vi "SP_OEE_2_test.vi"() -> ()   [LabVIEW 2017] (continued)
                        n1245 = Decimal String To Number(string=w6823) -> (number=w6842:i32[])  [unwired: 2 in, 1 out]
                        n1246 = Decimal String To Number(string=w6824) -> (number=w6843:i32[])  [unwired: 2 in, 1 out]
                        n1247 = Decimal String To Number(string=w6825) -> (number=w6838:i32[])  [unwired: 2 in, 1 out]
                        n1248 = Compound Arithmetic op=ADD(w6815, w6813, w6811, w6809, w6807) -> (w6818:dbl[])
                        n1249 = Build Array(w6816) -> (w6837:string[][])
                        n1250 = Build Array(w6814) -> (w6836:string[][])
                        n1251 = Build Array(w6812) -> (w6835:string[][])
                        n1252 = Build Array(w6810) -> (w6834:string[][])
                        n1253 = Build Array(w6808) -> (w6833:string[][])
                        n1254 = Number To Fractional String(number=w6818, precision (6)=i16 2) -> (F-format string=w6817:string[])  [unwired: 2 in]
                        n1255 = Compound Arithmetic op=ADD(w6840, w6841, w6842, w6843, w6838) -> (w6844:i32[])
                        n1256 = Transpose 2D Array(2D array=w6837) -> (transposed array=w6831:string[][])
                        n1257 = Transpose 2D Array(2D array=w6836) -> (transposed array=w6830:string[][])
                        n1258 = Transpose 2D Array(2D array=w6835) -> (transposed array=w6829:string[][])
                        n1259 = Transpose 2D Array(2D array=w6834) -> (transposed array=w6828:string[][])
                        n1260 = Transpose 2D Array(2D array=w6833) -> (transposed array=w6827:string[][])
                        n1261 = Number To Decimal String(number=w6844) -> (decimal integer string=w6839:string[])  [unwired: 1 in]
                        n1262 = Build Array(w6817) -> (w6820:string[][])
                        n1263 = Transpose 2D Array(2D array=w6820) -> (transposed array=w6826:string[][])
                      }
                      frame #7 {
                        w6849 = string[] [""]
                        n1264 = Insert Into Array(array=w6857, index (col)=1 ("disabled index (col)"), new element #1=w6849, new element #2=w6849, new element #3=w6849, new element #4=w6849, new element #5=w6849, new element #6=w6849, new element #7=w6848, new element #8=w6847, new element #9=w6849, new element #10=w6849, new element #11=w6850, new element #12=w6851) -> (w6853:string[][])  [unwired: 1 in]
                        n1265 = call "flot graph for month n year.vi"("BD Date"=w6854, "error in (no error)"=w6856, "Count total"=w6850) -> ("error out"=w6855:errorcluster, "Run-Time Status"=w6852:cluster{"Array 2":timestamp[], dbl[]})  [unwired: 7 in]
                        n1266 = local write "Run-Time Status"(w6852) -> ()
                        n1267 = local write "Table"(w6853) -> ()
                      }
                    }
                  }
                  frame "2" {
                    n1268 = flat-sequence {
                      tunnel: w6869 -> [w6983]
                      tunnel: w6868 -> [w6981]
                      tunnel: [w6967] -> w6959
                      tunnel: [w6982] -> w6958
                      tunnel: w6867 -> [_]
                      tunnel: [w6986] -> w6957
                      tunnel: [w6966] -> w6956
                      tunnel: [w6965] -> w6955
                      tunnel: [w6964] -> w6954
                      tunnel: w6866 -> [w6966]
                      tunnel: w6865 -> [w6965]
                      tunnel: ["Where BREAKDOWN_DATE between '%s'and '%s' and BREAKDOWN_STK_HOLD_ID ='%d' and  SHIFT_ID = '%d' "] -> w6953
                      tunnel: [w6964] -> w6952
                      tunnel: w6864 -> [w6960]
                      tunnel: [w6960] -> w6863
                      tunnel: w6959 -> [w7047]
                      tunnel: w6958 -> [w7049]
                      tunnel: w6957 -> [w7045]
                      tunnel: w6956 -> [w7044]
                      tunnel: w6955 -> [w7043]
                      tunnel: [w7046] -> w6951
                      tunnel: [w7048] -> w6950
                      tunnel: [w7045] -> w6949
                      tunnel: [w7035] -> w6948
                      tunnel: [w7041] -> w6947
                      tunnel: [w7044] -> w6946
                      tunnel: [w7043] -> w6945
                      tunnel: w6954 -> [w7040]
                      tunnel: [w7040] -> w6944
                      tunnel: w6953 -> [w7037]
                      tunnel: [w7037] -> w6943
                      tunnel: [w7036] -> w6942
                      tunnel: w6952 -> [w7036]
                      tunnel: w6863 -> [w7034]
                      tunnel: [w7033] -> w6862
                      tunnel: w6951 -> [w7079]
                      tunnel: w6950 -> [w7077]
                      tunnel: w6949 -> [w7082]
                      tunnel: w6948 -> [w7081]
                      tunnel: w6947 -> [w7080]
                      tunnel: w6946 -> [w7075]
                      tunnel: w6945 -> [w7074]
                      tunnel: [w7082] -> w6941
                      tunnel: [w7081] -> w6940
                      tunnel: [w7080] -> w6939
                      tunnel: [w7078] -> w6938
                      tunnel: [w7072] -> w6937
                      tunnel: [w7071] -> w6936
                      tunnel: [w7076] -> w6935
                      tunnel: [w7075] -> w6934
                      tunnel: [w7074] -> w6933
                      tunnel: w6944 -> [w7070]
                      tunnel: [w7070] -> w6932
                      tunnel: w6943 -> [w7067]
                      tunnel: [w7067] -> w6931
                      tunnel: [w7066] -> w6930
                      tunnel: w6942 -> [w7066]
                      tunnel: w6862 -> [w7065]
                      tunnel: [w7064] -> w6861
                      tunnel: w6941 -> [w7117]
                      tunnel: w6940 -> [w7116]
                      tunnel: w6939 -> [w7115]
                      tunnel: w6938 -> [w7112]
                      tunnel: w6937 -> [w7114]
                      tunnel: w6936 -> [w7113]
                      tunnel: w6935 -> [w7110]
                      tunnel: w6934 -> [w7108]
                      tunnel: w6933 -> [w7107]
                      tunnel: [w7117] -> w6929
                      tunnel: [w7116] -> w6928
                      tunnel: [w7115] -> w6927
                      tunnel: [w7114] -> w6926
                      tunnel: [w7113] -> w6925
                      tunnel: [w7111] -> w6924
                      tunnel: [w7105] -> w6923
                      tunnel: [w7104] -> w6922
                      tunnel: [w7109] -> w6921
                      tunnel: [w7108] -> w6920
                      tunnel: [w7107] -> w6919
                      tunnel: w6932 -> [w7103]
                      tunnel: [w7103] -> w6918
                      tunnel: w6931 -> [w7100]
                      tunnel: [w7100] -> w6917
                      tunnel: [w7099] -> w6916
                      tunnel: w6930 -> [w7099]
                      tunnel: w6861 -> [w7098]
                      tunnel: [w7097] -> w6860
                      tunnel: w6929 -> [w7154]
                      tunnel: w6928 -> [w7153]
                      tunnel: w6927 -> [w7152]
                      tunnel: w6926 -> [w7151]
                      tunnel: w6925 -> [w7150]
                      tunnel: w6924 -> [w7147]
                      tunnel: w6923 -> [w7149]
                      tunnel: w6922 -> [w7148]
                      tunnel: w6921 -> [w7146]
                      tunnel: w6920 -> [w7143]
                      tunnel: w6919 -> [w7142]
                      tunnel: [w7154] -> w6915
                      tunnel: [w7153] -> w6914
                      tunnel: [w7152] -> w6913
                      tunnel: [w7151] -> w6912
                      tunnel: [w7150] -> w6911
                      tunnel: [w7149] -> w6910
                      tunnel: [w7148] -> w6909
                      tunnel: [w7145] -> w6908
                      tunnel: [w7144] -> w6907
                      tunnel: [w7140] -> w6906
                      tunnel: [w7139] -> w6905
                      tunnel: [w7143] -> w6904
                      tunnel: [w7142] -> w6903
                      tunnel: w6918 -> [w7138]
                      tunnel: [w7138] -> w6902
                      tunnel: w6917 -> [w7135]
                      tunnel: [w7135] -> w6901
                      tunnel: [w7134] -> w6900
                      tunnel: w6916 -> [w7134]
                      tunnel: w6860 -> [w7132]
                      tunnel: w6915 -> [w7177]
                      tunnel: w6914 -> [w7176]
                      tunnel: w6913 -> [w7175]
                      tunnel: w6912 -> [w7174]
                      tunnel: w6911 -> [w7173]
                      tunnel: w6910 -> [w7172]
                      tunnel: w6909 -> [w7171]
                      tunnel: w6908 -> [w7166]
                      tunnel: w6907 -> [w7168]
                      tunnel: w6906 -> [w7170]
                      tunnel: w6905 -> [w7169]
                      tunnel: w6904 -> [w7163]
                      tunnel: w6903 -> [w7164]
                      tunnel: [w7177] -> w6899
                      tunnel: [w7176] -> w6898
                      tunnel: [w7175] -> w6897
                      tunnel: [w7174] -> w6896
                      tunnel: [w7173] -> w6895
                      tunnel: [w7172] -> w6894
                      tunnel: [w7171] -> w6893
                      tunnel: [w7170] -> w6892
                      tunnel: [w7169] -> w6891
                      tunnel: [w7167] -> w6890
                      tunnel: [w7165] -> w6889
                      tunnel: [w7161] -> w6888
                      tunnel: [w7159] -> w6887
                      tunnel: w6902 -> [w7160]
                      tunnel: w6901 -> [w7156]
                      tunnel: [w7155] -> w6886
                      tunnel: w6900 -> [w7155]
                      tunnel: w6899 -> [w7216]
                      tunnel: w6898 -> [w7209]
                      tunnel: w6897 -> [w7200]
                      tunnel: w6896 -> [w7208]
                      tunnel: w6895 -> [w7198]
                      tunnel: w6894 -> [w7207]
                      tunnel: w6893 -> [w7196]
                      tunnel: w6892 -> [w7206]
                      tunnel: w6891 -> [w7194]
                      tunnel: w6890 -> [w7230]
                      tunnel: w6889 -> [w7229]
                      tunnel: w6888 -> [w7205]
                      tunnel: w6887 -> [w7192]
                      tunnel: [w7230] -> w6885
                      tunnel: [w7229] -> w6884
                      tunnel: [w7223] -> w6883
                      tunnel: [w7216] -> w6882
                      tunnel: [w7215] -> w6881
                      tunnel: [w7214] -> w6880
                      tunnel: [w7213] -> w6879
                      tunnel: [w7212] -> w6878
                      tunnel: [w7211] -> w6877
                      tunnel: [w7210] -> w6876
                      tunnel: [w7209] -> w6875
                      tunnel: [w7208] -> w6874
                      tunnel: [w7207] -> w6873
                      tunnel: [w7206] -> w6872
                      tunnel: [w7205] -> w6871
                      tunnel: [w7190] -> w6870
                      tunnel: w6886 -> [w7190]
                      tunnel: [w7243] -> _
                      tunnel: [w7239] -> _
                      tunnel: w6885 -> [w7240]
                      tunnel: w6884 -> [w7243]
                      tunnel: w6883 -> [w7234]
                      tunnel: w6882 -> [w7241]
                      tunnel: w6881 -> [_]
                      tunnel: w6880 -> [_]
                      tunnel: w6879 -> [_]
                      tunnel: w6878 -> [w7231]
                      tunnel: w6877 -> [_]
                      tunnel: w6876 -> [w7235]
                      tunnel: w6875 -> [_]
                      tunnel: w6874 -> [_]
                      tunnel: w6873 -> [_]
                      tunnel: w6872 -> [w7232]
                      tunnel: w6871 -> [_]
                      tunnel: w6870 -> [w7238]
                      frame #0 {
                        w6974 = "%Y-%m-%d" ("time format string (%c)")
                        n1269 = Decimal String To Number(string=w6960) -> (number=w6961:i32)  [unwired: 2 in, 1 out]
                        n1270 = property on="Table" class="Tbl (strict)"("Visible"=TRUE) -> ()  [unwired: 2 in, 2 out]
                        n1271 = Format Date/Time String(time format string (%c)=w6974, seconds (now)=w6966) -> (date/time string=w6975:string)  [unwired: 1 in]
                        n1272 = Format Date/Time String(time format string (%c)=w6974, seconds (now)=w6965) -> (date/time string=w6973:string)  [unwired: 1 in]
                        n1273 = Format Into String(format string="Where BREAKDOWN_DATE between '%s' and '%s' and  SHIFT_ID = '%d'  ", w6975, w6973, w6961) -> (resulting string=w6972:string)  [unwired: 2 in, 1 out]
                        n1274 = call <vilib>:"DB Tools Select Data.vi"("condition"=w6972, "error in (no error)"=w6981, "columns"=string[] ["BREAKDOWN_DATE"], "table"="STATION_1_LOG_HISTORY", "connection reference"=w6983) -> ("error out"=w6968:errorcluster, "data"=w6971:variant[][], "connection reference out"=w6982:T2)  [unwired: 1 in]
                        n1275 = property on="Table 2" class="Tbl (strict)"("Visible"=FALSE) -> ()  [unwired: 2 in, 2 out]
                        n1276 = xnode "Database Variant To Data"("database variant"=w6971, "error in (no error)"=w6968, "type"=string[][] [] ("Elements Found")) -> ("data"=w6969:string[][], "error out"=w6967:errorcluster)
                        n1277 = Index Array(array=w6969, index (col)=0 ("disabled index (col)")) -> (element=w6977:string[])  [unwired: 1 in]
                        n1278 = call "Search_1d_array_element.vi"("Count in"=string[] [] ("Elements Found"), "BD Date"=w6977, "Elements Found in"=string[] [] ("Elements Found")) -> ("Elements Found out"=w6964:string[])  [unwired: 4 in, 2 out]
                        n1279 = Build Array(w6964) -> (w6987:string[][])
                        n1280 = Transpose 2D Array(2D array=w6987) -> (transposed array=w6986:string[][])
                      }
                      frame #1 {
                        n1281 = disable-structure shown="Enabled" {
                          disable-tunnel: w7049 -> [w7060 w7062]
                          disable-tunnel: [w7059 w7062] -> w7048
                          disable-tunnel: w7047 -> [w7058 w7063]
                          disable-tunnel: [w7057 w7063] -> w7046
                          disable-tunnel: w7044 -> [w7055 _]
                          disable-tunnel: w7043 -> [w7054 _]
                          disable-tunnel: [w7053 _] -> w7042
                          disable-tunnel: [w7052 _] -> w7039
                          disable-tunnel: w7037 -> [w7051 _]
                          disable-tunnel: w7034 -> [w7050 w7061]
                          disable-tunnel: [_ w7061] -> w7033
                          frame Disabled {
                            n1282 = call "Stack_holderwise_total_bd_count_&_duration_2.vi"("Refnum in"=w7060, "BREAKDOWN_STK_HOLD_ID"=1, "condition"=w7051, "Form Date"=w7055, "To Date"=w7054, "error in (no error)"=w7058, "Shift"=w7050) -> ("Refnum out"=w7059:T2, "Count out"=w7053:string[], "appended array"=w7052:dbl[], "error out"=w7057:errorcluster)  [unwired: 5 in]
                          }
                          frame Enabled {
                          }
                        }
                        n1283 = call "NUMERIC TO STRING.vi"("appended array"=w7039) -> ("Array"=w7038:string[])  [unwired: 4 in]
                        n1284 = call "Insert_empty_element_with_zero.vi"("searched date"=w7042, "fixed date"=w7040) -> ("O/P"=w7035:string[])  [unwired: 9 in]
                        n1285 = call "Insert_empty_element_with_zero.vi"("searched date"=w7038, "fixed date"=w7040) -> ("O/P"=w7041:string[])  [unwired: 9 in]
                      }
                      frame #2 {
                        n1286 = disable-structure shown="Enabled" {
                          disable-tunnel: w7079 -> [w7093 w7095]
                          disable-tunnel: [w7092 w7095] -> w7078
                          disable-tunnel: w7077 -> [w7091 w7096]
                          disable-tunnel: [w7090 w7096] -> w7076
                          disable-tunnel: w7075 -> [w7089 _]
                          disable-tunnel: w7074 -> [w7088 _]
                          disable-tunnel: [w7087 _] -> w7073
                          disable-tunnel: [w7086 _] -> w7069
                          disable-tunnel: w7067 -> [w7085 _]
                          disable-tunnel: w7065 -> [w7083 w7094]
                          disable-tunnel: [_ w7094] -> w7064
                          frame Disabled {
                            n1287 = call "Stack_holderwise_total_bd_count_&_duration_2.vi"("Refnum in"=w7091, "BREAKDOWN_STK_HOLD_ID"=2, "condition"=w7085, "Form Date"=w7089, "To Date"=w7088, "error in (no error)"=w7093, "Shift"=w7083) -> ("Refnum out"=w7090:T2, "Count out"=w7087:string[], "appended array"=w7086:dbl[], "error out"=w7092:errorcluster)  [unwired: 5 in]
                          }
                          frame Enabled {
                          }
                        }
                        n1288 = call "Insert_empty_element_with_zero.vi"("searched date"=w7073, "fixed date"=w7070) -> ("O/P"=w7072:string[])  [unwired: 9 in]
                        n1289 = call "NUMERIC TO STRING.vi"("appended array"=w7069) -> ("Array"=w7068:string[])  [unwired: 4 in]
                        n1290 = call "Insert_empty_element_with_zero.vi"("searched date"=w7068, "fixed date"=w7070) -> ("O/P"=w7071:string[])  [unwired: 9 in]
                      }
                      frame #3 {
                        n1291 = disable-structure shown="Enabled" {
                          disable-tunnel: w7112 -> [w7128 w7130]
                          disable-tunnel: [w7127 w7130] -> w7111
                          disable-tunnel: w7110 -> [w7126 w7131]
                          disable-tunnel: [w7125 w7131] -> w7109
                          disable-tunnel: w7108 -> [w7124 _]
                          disable-tunnel: w7107 -> [w7123 _]
                          disable-tunnel: [w7122 _] -> w7106
                          disable-tunnel: [w7121 _] -> w7102
                          disable-tunnel: w7100 -> [w7120 _]
                          disable-tunnel: w7098 -> [w7118 w7129]
                          disable-tunnel: [_ w7129] -> w7097
                          frame Disabled {
                            n1292 = call "Stack_holderwise_total_bd_count_&_duration_2.vi"("Refnum in"=w7126, "BREAKDOWN_STK_HOLD_ID"=3, "condition"=w7120, "Form Date"=w7124, "To Date"=w7123, "error in (no error)"=w7128, "Shift"=w7118) -> ("Refnum out"=w7125:T2, "Count out"=w7122:string[], "appended array"=w7121:dbl[], "error out"=w7127:errorcluster)  [unwired: 5 in]
                          }
                          frame Enabled {
                          }
                        }
                        n1293 = call "Insert_empty_element_with_zero.vi"("searched date"=w7106, "fixed date"=w7103) -> ("O/P"=w7105:string[])  [unwired: 9 in]
                        n1294 = call "NUMERIC TO STRING.vi"("appended array"=w7102) -> ("Array"=w7101:string[])  [unwired: 4 in]
                        n1295 = call "Insert_empty_element_with_zero.vi"("searched date"=w7101, "fixed date"=w7103) -> ("O/P"=w7104:string[])  [unwired: 9 in]
                      }
                      frame #4 {
                        n1296 = call "Stack_holderwise_total_bd_count_&_duration_2.vi"("Refnum in"=w7146, "BREAKDOWN_STK_HOLD_ID"=4, "condition"=w7135, "Form Date"=w7143, "To Date"=w7142, "error in (no error)"=w7147, "Shift"=w7132) -> ("Refnum out"=w7145:T2, "Count out"=w7141:string[], "appended array"=w7137:dbl[], "error out"=w7144:errorcluster)  [unwired: 5 in]
                        n1297 = call "Insert_empty_element_with_zero.vi"("searched date"=w7141, "fixed date"=w7138) -> ("O/P"=w7140:string[])  [unwired: 9 in]
                        n1298 = call "NUMERIC TO STRING.vi"("appended array"=w7137) -> ("Array"=w7136:string[])  [unwired: 4 in]
                        n1299 = call "Insert_empty_element_with_zero.vi"("searched date"=w7136, "fixed date"=w7138) -> ("O/P"=w7139:string[])  [unwired: 9 in]
                      }
                      frame #5 {
                        n1300 = disable-structure shown="Enabled" {
                          disable-tunnel: w7168 -> [w7186 w7189]
                          disable-tunnel: [w7185 w7189] -> w7167
                          disable-tunnel: w7166 -> [w7184 w7188]
                          disable-tunnel: [w7183 w7188] -> w7165
                          disable-tunnel: w7164 -> [w7182 _]
                          disable-tunnel: w7163 -> [w7181 _]
                          disable-tunnel: [w7180 _] -> w7162
                          disable-tunnel: [w7179 _] -> w7158
                          disable-tunnel: w7156 -> [w7178 _]
                          frame Disabled {
                            n1301 = call "Stack_holderwise_total_bd_count_&_duration.vi"("Refnum in"=w7184, "BREAKDOWN_STK_HOLD_ID"=5, "condition"=w7178, "Form Date"=w7181, "To Date"=w7182, "error in (no error)"=w7186) -> ("Refnum out"=w7183:T2, "Count out"=w7180:string[], "appended array"=w7179:dbl[], "error out"=w7185:errorcluster)  [unwired: 6 in]
                          }
                          frame Enabled {
                          }
                        }
                        n1302 = call "NUMERIC TO STRING.vi"("appended array"=w7158) -> ("Array"=w7157:string[])  [unwired: 4 in]
                        n1303 = call "Insert_empty_element_with_zero.vi"("searched date"=w7162, "fixed date"=w7160) -> ("O/P"=w7161:string[])  [unwired: 9 in]
                        n1304 = call "Insert_empty_element_with_zero.vi"("searched date"=w7157, "fixed date"=w7160) -> ("O/P"=w7159:string[])  [unwired: 9 in]
                      }
                      frame #6 {
                        n1305 = call "String to numeric.vi"("Array"=w7200) -> ("Array 2"=w7199:dbl[])  [unwired: 4 in]
                        n1306 = call "String to numeric.vi"("Array"=w7198) -> ("Array 2"=w7197:dbl[])  [unwired: 4 in]
                        n1307 = call "String to numeric.vi"("Array"=w7196) -> ("Array 2"=w7195:dbl[])  [unwired: 4 in]
                        n1308 = call "String to numeric.vi"("Array"=w7194) -> ("Array 2"=w7193:dbl[])  [unwired: 4 in]
                        n1309 = call "String to numeric.vi"("Array"=w7192) -> ("Array 2"=w7191:dbl[])  [unwired: 4 in]
                        n1310 = Decimal String To Number(string=w7205) -> (number=w7224:i32[])  [unwired: 2 in, 1 out]
                        n1311 = Decimal String To Number(string=w7206) -> (number=w7225:i32[])  [unwired: 2 in, 1 out]
                        n1312 = Decimal String To Number(string=w7207) -> (number=w7226:i32[])  [unwired: 2 in, 1 out]
                        n1313 = Decimal String To Number(string=w7208) -> (number=w7227:i32[])  [unwired: 2 in, 1 out]
                        n1314 = Decimal String To Number(string=w7209) -> (number=w7222:i32[])  [unwired: 2 in, 1 out]
                        n1315 = Compound Arithmetic op=ADD(w7199, w7197, w7195, w7193, w7191) -> (w7202:dbl[])
                        n1316 = Build Array(w7200) -> (w7221:string[][])
                        n1317 = Build Array(w7198) -> (w7220:string[][])
                        n1318 = Build Array(w7196) -> (w7219:string[][])
                        n1319 = Build Array(w7194) -> (w7218:string[][])
                        n1320 = Build Array(w7192) -> (w7217:string[][])
                        n1321 = Number To Fractional String(number=w7202, precision (6)=i16 2) -> (F-format string=w7201:string[])  [unwired: 2 in]
                        n1322 = Compound Arithmetic op=ADD(w7224, w7225, w7226, w7227, w7222) -> (w7228:i32[])
                        n1323 = Transpose 2D Array(2D array=w7221) -> (transposed array=w7215:string[][])
                        n1324 = Transpose 2D Array(2D array=w7220) -> (transposed array=w7214:string[][])
                        n1325 = Transpose 2D Array(2D array=w7219) -> (transposed array=w7213:string[][])
                        n1326 = Transpose 2D Array(2D array=w7218) -> (transposed array=w7212:string[][])
                        n1327 = Transpose 2D Array(2D array=w7217) -> (transposed array=w7211:string[][])
                        n1328 = Number To Decimal String(number=w7228) -> (decimal integer string=w7223:string[])  [unwired: 1 in]
                        n1329 = Build Array(w7201) -> (w7204:string[][])
                        n1330 = Transpose 2D Array(2D array=w7204) -> (transposed array=w7210:string[][])
                      }
                      frame #7 {
                        w7233 = string[] [""]
                        n1331 = Insert Into Array(array=w7241, index (col)=1 ("disabled index (col)"), new element #1=w7233, new element #2=w7233, new element #3=w7233, new element #4=w7233, new element #5=w7233, new element #6=w7233, new element #7=w7232, new element #8=w7231, new element #9=w7233, new element #10=w7233, new element #11=w7234, new element #12=w7235) -> (w7237:string[][])  [unwired: 1 in]
                        n1332 = call "flot graph for month n year.vi"("BD Date"=w7238, "error in (no error)"=w7240, "Count total"=w7234) -> ("error out"=w7239:errorcluster, "Run-Time Status"=w7236:cluster{"Array 2":timestamp[], dbl[]})  [unwired: 7 in]
                        n1333 = local write "Run-Time Status"(w7236) -> ()
                        n1334 = local write "Table"(w7237) -> ()
                      }
                    }
                  }
                  frame "3" {
                    n1335 = flat-sequence {
                      tunnel: w7253 -> [w7367]
                      tunnel: w7252 -> [w7365]
                      tunnel: [w7351] -> w7343
                      tunnel: [w7366] -> w7342
                      tunnel: w7251 -> [_]
                      tunnel: [w7370] -> w7341
                      tunnel: [w7350] -> w7340
                      tunnel: [w7349] -> w7339
                      tunnel: [w7348] -> w7338
                      tunnel: w7250 -> [w7350]
                      tunnel: w7249 -> [w7349]
                      tunnel: ["Where BREAKDOWN_DATE between '%s'and '%s' and BREAKDOWN_STK_HOLD_ID ='%d' and  SHIFT_ID = '%d' "] -> w7337
                      tunnel: [w7348] -> w7336
                      tunnel: w7248 -> [w7344]
                      tunnel: [w7344] -> w7247
                      tunnel: w7343 -> [w7431]
                      tunnel: w7342 -> [w7433]
                      tunnel: w7341 -> [w7429]
                      tunnel: w7340 -> [w7428]
                      tunnel: w7339 -> [w7427]
                      tunnel: [w7430] -> w7335
                      tunnel: [w7432] -> w7334
                      tunnel: [w7429] -> w7333
                      tunnel: [w7419] -> w7332
                      tunnel: [w7425] -> w7331
                      tunnel: [w7428] -> w7330
                      tunnel: [w7427] -> w7329
                      tunnel: w7338 -> [w7424]
                      tunnel: [w7424] -> w7328
                      tunnel: w7337 -> [w7421]
                      tunnel: [w7421] -> w7327
                      tunnel: [w7420] -> w7326
                      tunnel: w7336 -> [w7420]
                      tunnel: w7247 -> [w7418]
                      tunnel: [w7417] -> w7246
                      tunnel: w7335 -> [w7463]
                      tunnel: w7334 -> [w7461]
                      tunnel: w7333 -> [w7466]
                      tunnel: w7332 -> [w7465]
                      tunnel: w7331 -> [w7464]
                      tunnel: w7330 -> [w7459]
                      tunnel: w7329 -> [w7458]
                      tunnel: [w7466] -> w7325
                      tunnel: [w7465] -> w7324
                      tunnel: [w7464] -> w7323
                      tunnel: [w7462] -> w7322
                      tunnel: [w7456] -> w7321
                      tunnel: [w7455] -> w7320
                      tunnel: [w7460] -> w7319
                      tunnel: [w7459] -> w7318
                      tunnel: [w7458] -> w7317
                      tunnel: w7328 -> [w7454]
                      tunnel: [w7454] -> w7316
                      tunnel: w7327 -> [w7451]
                      tunnel: [w7451] -> w7315
                      tunnel: [w7450] -> w7314
                      tunnel: w7326 -> [w7450]
                      tunnel: w7246 -> [w7449]
                      tunnel: [w7448] -> w7245
                      tunnel: w7325 -> [w7501]
                      tunnel: w7324 -> [w7500]
                      tunnel: w7323 -> [w7499]
                      tunnel: w7322 -> [w7496]
                      tunnel: w7321 -> [w7498]
                      tunnel: w7320 -> [w7497]
                      tunnel: w7319 -> [w7494]
                      tunnel: w7318 -> [w7492]
                      tunnel: w7317 -> [w7491]
                      tunnel: [w7501] -> w7313
                      tunnel: [w7500] -> w7312
                      tunnel: [w7499] -> w7311
                      tunnel: [w7498] -> w7310
                      tunnel: [w7497] -> w7309
                      tunnel: [w7495] -> w7308
                      tunnel: [w7489] -> w7307
                      tunnel: [w7488] -> w7306
                      tunnel: [w7493] -> w7305
                      tunnel: [w7492] -> w7304
                      tunnel: [w7491] -> w7303
                      tunnel: w7316 -> [w7487]
                      tunnel: [w7487] -> w7302
                      tunnel: w7315 -> [w7484]
                      tunnel: [w7484] -> w7301
                      tunnel: [w7483] -> w7300
                      tunnel: w7314 -> [w7483]
                      tunnel: w7245 -> [w7482]
                      tunnel: [w7481] -> w7244
                      tunnel: w7313 -> [w7538]
                      tunnel: w7312 -> [w7537]
                      tunnel: w7311 -> [w7536]
                      tunnel: w7310 -> [w7535]
                      tunnel: w7309 -> [w7534]
                      tunnel: w7308 -> [w7531]
                      tunnel: w7307 -> [w7533]
                      tunnel: w7306 -> [w7532]
                      tunnel: w7305 -> [w7530]
                      tunnel: w7304 -> [w7527]
                      tunnel: w7303 -> [w7526]
                      tunnel: [w7538] -> w7299
                      tunnel: [w7537] -> w7298
                      tunnel: [w7536] -> w7297
                      tunnel: [w7535] -> w7296
                      tunnel: [w7534] -> w7295
                      tunnel: [w7533] -> w7294
                      tunnel: [w7532] -> w7293
                      tunnel: [w7529] -> w7292
                      tunnel: [w7528] -> w7291
                      tunnel: [w7524] -> w7290
                      tunnel: [w7523] -> w7289
                      tunnel: [w7527] -> w7288
                      tunnel: [w7526] -> w7287
                      tunnel: w7302 -> [w7522]
                      tunnel: [w7522] -> w7286
                      tunnel: w7301 -> [w7519]
                      tunnel: [w7519] -> w7285
                      tunnel: [w7518] -> w7284
                      tunnel: w7300 -> [w7518]
                      tunnel: w7244 -> [w7516]
                      tunnel: w7299 -> [w7561]
                      tunnel: w7298 -> [w7560]
                      tunnel: w7297 -> [w7559]
                      tunnel: w7296 -> [w7558]
                      tunnel: w7295 -> [w7557]
                      tunnel: w7294 -> [w7556]
                      tunnel: w7293 -> [w7555]
                      tunnel: w7292 -> [w7550]
                      tunnel: w7291 -> [w7552]
                      tunnel: w7290 -> [w7554]
                      tunnel: w7289 -> [w7553]
                      tunnel: w7288 -> [w7547]
                      tunnel: w7287 -> [w7548]
                      tunnel: [w7561] -> w7283
                      tunnel: [w7560] -> w7282
                      tunnel: [w7559] -> w7281
                      tunnel: [w7558] -> w7280
                      tunnel: [w7557] -> w7279
                      tunnel: [w7556] -> w7278
                      tunnel: [w7555] -> w7277
                      tunnel: [w7554] -> w7276
                      tunnel: [w7553] -> w7275
                      tunnel: [w7551] -> w7274
                      tunnel: [w7549] -> w7273
                      tunnel: [w7545] -> w7272
                      tunnel: [w7543] -> w7271
                      tunnel: w7286 -> [w7544]
                      tunnel: w7285 -> [w7540]
                      tunnel: [w7539] -> w7270
                      tunnel: w7284 -> [w7539]
                      tunnel: w7283 -> [w7600]
                      tunnel: w7282 -> [w7593]
                      tunnel: w7281 -> [w7584]
                      tunnel: w7280 -> [w7592]
                      tunnel: w7279 -> [w7582]
                      tunnel: w7278 -> [w7591]
                      tunnel: w7277 -> [w7580]
                      tunnel: w7276 -> [w7590]
                      tunnel: w7275 -> [w7578]
                      tunnel: w7274 -> [w7614]
                      tunnel: w7273 -> [w7613]
                      tunnel: w7272 -> [w7589]
                      tunnel: w7271 -> [w7576]
                      tunnel: [w7614] -> w7269
                      tunnel: [w7613] -> w7268
                      tunnel: [w7607] -> w7267
                      tunnel: [w7600] -> w7266
                      tunnel: [w7599] -> w7265
                      tunnel: [w7598] -> w7264
                      tunnel: [w7597] -> w7263
                      tunnel: [w7596] -> w7262
                      tunnel: [w7595] -> w7261
                      tunnel: [w7594] -> w7260
                      tunnel: [w7593] -> w7259
                      tunnel: [w7592] -> w7258
                      tunnel: [w7591] -> w7257
                      tunnel: [w7590] -> w7256
                      tunnel: [w7589] -> w7255
                      tunnel: [w7574] -> w7254
                      tunnel: w7270 -> [w7574]
                      tunnel: [w7627] -> _
                      tunnel: [w7623] -> _
                      tunnel: w7269 -> [w7624]
                      tunnel: w7268 -> [w7627]
                      tunnel: w7267 -> [w7618]
                      tunnel: w7266 -> [w7625]
                      tunnel: w7265 -> [_]
                      tunnel: w7264 -> [_]
                      tunnel: w7263 -> [_]
                      tunnel: w7262 -> [w7615]
                      tunnel: w7261 -> [_]
                      tunnel: w7260 -> [w7619]
                      tunnel: w7259 -> [_]
                      tunnel: w7258 -> [_]
                      tunnel: w7257 -> [_]
                      tunnel: w7256 -> [w7616]
                      tunnel: w7255 -> [_]
                      tunnel: w7254 -> [w7622]
                      frame #0 {
                        w7358 = "%Y-%m-%d" ("time format string (%c)")
                        n1336 = Decimal String To Number(string=w7344) -> (number=w7345:i32)  [unwired: 2 in, 1 out]
                        n1337 = property on="Table" class="Tbl (strict)"("Visible"=TRUE) -> ()  [unwired: 2 in, 2 out]
                        n1338 = Format Date/Time String(time format string (%c)=w7358, seconds (now)=w7350) -> (date/time string=w7359:string)  [unwired: 1 in]
                        n1339 = Format Date/Time String(time format string (%c)=w7358, seconds (now)=w7349) -> (date/time string=w7357:string)  [unwired: 1 in]
                        n1340 = Format Into String(format string="Where BREAKDOWN_DATE between '%s' and '%s' and  SHIFT_ID = '%d'  ", w7359, w7357, w7345) -> (resulting string=w7356:string)  [unwired: 2 in, 1 out]
                        n1341 = call <vilib>:"DB Tools Select Data.vi"("condition"=w7356, "error in (no error)"=w7365, "columns"=string[] ["BREAKDOWN_DATE"], "table"="STATION_1_LOG_HISTORY", "connection reference"=w7367) -> ("error out"=w7352:errorcluster, "data"=w7355:variant[][], "connection reference out"=w7366:T2)  [unwired: 1 in]
                        n1342 = property on="Table 2" class="Tbl (strict)"("Visible"=FALSE) -> ()  [unwired: 2 in, 2 out]
                        n1343 = xnode "Database Variant To Data"("database variant"=w7355, "error in (no error)"=w7352, "type"=string[][] [] ("Elements Found")) -> ("data"=w7353:string[][], "error out"=w7351:errorcluster)
                        n1344 = Index Array(array=w7353, index (col)=0 ("disabled index (col)")) -> (element=w7361:string[])  [unwired: 1 in]
                        n1345 = call "Search_1d_array_element.vi"("Count in"=string[] [] ("Elements Found"), "BD Date"=w7361, "Elements Found in"=string[] [] ("Elements Found")) -> ("Elements Found out"=w7348:string[])  [unwired: 4 in, 2 out]
                        n1346 = Build Array(w7348) -> (w7371:string[][])
                        n1347 = Transpose 2D Array(2D array=w7371) -> (transposed array=w7370:string[][])
                      }
                      frame #1 {
                        n1348 = disable-structure shown="Enabled" {
                          disable-tunnel: w7433 -> [w7444 w7446]
                          disable-tunnel: [w7443 w7446] -> w7432
                          disable-tunnel: w7431 -> [w7442 w7447]
                          disable-tunnel: [w7441 w7447] -> w7430
                          disable-tunnel: w7428 -> [w7439 _]
                          disable-tunnel: w7427 -> [w7438 _]
                          disable-tunnel: [w7437 _] -> w7426
                          disable-tunnel: [w7436 _] -> w7423
                          disable-tunnel: w7421 -> [w7435 _]
                          disable-tunnel: w7418 -> [w7434 w7445]
                          disable-tunnel: [_ w7445] -> w7417
                          frame Disabled {
                            n1349 = call "Stack_holderwise_total_bd_count_&_duration_2.vi"("Refnum in"=w7444, "BREAKDOWN_STK_HOLD_ID"=1, "condition"=w7435, "Form Date"=w7439, "To Date"=w7438, "error in (no error)"=w7442, "Shift"=w7434) -> ("Refnum out"=w7443:T2, "Count out"=w7437:string[], "appended array"=w7436:dbl[], "error out"=w7441:errorcluster)  [unwired: 5 in]
                          }
                          frame Enabled {
                          }
                        }
                        n1350 = call "NUMERIC TO STRING.vi"("appended array"=w7423) -> ("Array"=w7422:string[])  [unwired: 4 in]
                        n1351 = call "Insert_empty_element_with_zero.vi"("searched date"=w7426, "fixed date"=w7424) -> ("O/P"=w7419:string[])  [unwired: 9 in]
                        n1352 = call "Insert_empty_element_with_zero.vi"("searched date"=w7422, "fixed date"=w7424) -> ("O/P"=w7425:string[])  [unwired: 9 in]
                      }
                      frame #2 {
                        n1353 = disable-structure shown="Enabled" {
                          disable-tunnel: w7463 -> [w7477 w7479]
                          disable-tunnel: [w7476 w7479] -> w7462
                          disable-tunnel: w7461 -> [w7475 w7480]
                          disable-tunnel: [w7474 w7480] -> w7460
                          disable-tunnel: w7459 -> [w7473 _]
                          disable-tunnel: w7458 -> [w7472 _]
                          disable-tunnel: [w7471 _] -> w7457
                          disable-tunnel: [w7470 _] -> w7453
                          disable-tunnel: w7451 -> [w7469 _]
                          disable-tunnel: w7449 -> [w7467 w7478]
                          disable-tunnel: [_ w7478] -> w7448
                          frame Disabled {
                            n1354 = call "Stack_holderwise_total_bd_count_&_duration_2.vi"("Refnum in"=w7475, "BREAKDOWN_STK_HOLD_ID"=2, "condition"=w7469, "Form Date"=w7473, "To Date"=w7472, "error in (no error)"=w7477, "Shift"=w7467) -> ("Refnum out"=w7474:T2, "Count out"=w7471:string[], "appended array"=w7470:dbl[], "error out"=w7476:errorcluster)  [unwired: 5 in]
                          }
                          frame Enabled {
                          }
                        }
                        n1355 = call "Insert_empty_element_with_zero.vi"("searched date"=w7457, "fixed date"=w7454) -> ("O/P"=w7456:string[])  [unwired: 9 in]
                        n1356 = call "NUMERIC TO STRING.vi"("appended array"=w7453) -> ("Array"=w7452:string[])  [unwired: 4 in]
                        n1357 = call "Insert_empty_element_with_zero.vi"("searched date"=w7452, "fixed date"=w7454) -> ("O/P"=w7455:string[])  [unwired: 9 in]
                      }
                      frame #3 {
                        n1358 = disable-structure shown="Enabled" {
                          disable-tunnel: w7496 -> [w7512 w7514]
                          disable-tunnel: [w7511 w7514] -> w7495
                          disable-tunnel: w7494 -> [w7510 w7515]
                          disable-tunnel: [w7509 w7515] -> w7493
                          disable-tunnel: w7492 -> [w7508 _]
                          disable-tunnel: w7491 -> [w7507 _]
                          disable-tunnel: [w7506 _] -> w7490
                          disable-tunnel: [w7505 _] -> w7486
                          disable-tunnel: w7484 -> [w7504 _]
                          disable-tunnel: w7482 -> [w7502 w7513]
                          disable-tunnel: [_ w7513] -> w7481
                          frame Disabled {
                            n1359 = call "Stack_holderwise_total_bd_count_&_duration_2.vi"("Refnum in"=w7510, "BREAKDOWN_STK_HOLD_ID"=3, "condition"=w7504, "Form Date"=w7508, "To Date"=w7507, "error in (no error)"=w7512, "Shift"=w7502) -> ("Refnum out"=w7509:T2, "Count out"=w7506:string[], "appended array"=w7505:dbl[], "error out"=w7511:errorcluster)  [unwired: 5 in]
                          }
                          frame Enabled {
                          }
                        }
                        n1360 = call "Insert_empty_element_with_zero.vi"("searched date"=w7490, "fixed date"=w7487) -> ("O/P"=w7489:string[])  [unwired: 9 in]
                        n1361 = call "NUMERIC TO STRING.vi"("appended array"=w7486) -> ("Array"=w7485:string[])  [unwired: 4 in]
                        n1362 = call "Insert_empty_element_with_zero.vi"("searched date"=w7485, "fixed date"=w7487) -> ("O/P"=w7488:string[])  [unwired: 9 in]
                      }
                      frame #4 {
                        n1363 = call "Stack_holderwise_total_bd_count_&_duration_2.vi"("Refnum in"=w7530, "BREAKDOWN_STK_HOLD_ID"=4, "condition"=w7519, "Form Date"=w7527, "To Date"=w7526, "error in (no error)"=w7531, "Shift"=w7516) -> ("Refnum out"=w7529:T2, "Count out"=w7525:string[], "appended array"=w7521:dbl[], "error out"=w7528:errorcluster)  [unwired: 5 in]
                        n1364 = call "Insert_empty_element_with_zero.vi"("searched date"=w7525, "fixed date"=w7522) -> ("O/P"=w7524:string[])  [unwired: 9 in]
                        n1365 = call "NUMERIC TO STRING.vi"("appended array"=w7521) -> ("Array"=w7520:string[])  [unwired: 4 in]
                        n1366 = call "Insert_empty_element_with_zero.vi"("searched date"=w7520, "fixed date"=w7522) -> ("O/P"=w7523:string[])  [unwired: 9 in]
                      }
                      frame #5 {
                        n1367 = disable-structure shown="Enabled" {
                          disable-tunnel: w7552 -> [w7570 w7573]
                          disable-tunnel: [w7569 w7573] -> w7551
                          disable-tunnel: w7550 -> [w7568 w7572]
                          disable-tunnel: [w7567 w7572] -> w7549
                          disable-tunnel: w7548 -> [w7566 _]
                          disable-tunnel: w7547 -> [w7565 _]
                          disable-tunnel: [w7564 _] -> w7546
                          disable-tunnel: [w7563 _] -> w7542
                          disable-tunnel: w7540 -> [w7562 _]
                          frame Disabled {
                            n1368 = call "Stack_holderwise_total_bd_count_&_duration.vi"("Refnum in"=w7568, "BREAKDOWN_STK_HOLD_ID"=5, "condition"=w7562, "Form Date"=w7565, "To Date"=w7566, "error in (no error)"=w7570) -> ("Refnum out"=w7567:T2, "Count out"=w7564:string[], "appended array"=w7563:dbl[], "error out"=w7569:errorcluster)  [unwired: 6 in]
                          }
                          frame Enabled {
                          }
                        }
                        n1369 = call "NUMERIC TO STRING.vi"("appended array"=w7542) -> ("Array"=w7541:string[])  [unwired: 4 in]
                        n1370 = call "Insert_empty_element_with_zero.vi"("searched date"=w7546, "fixed date"=w7544) -> ("O/P"=w7545:string[])  [unwired: 9 in]
                        n1371 = call "Insert_empty_element_with_zero.vi"("searched date"=w7541, "fixed date"=w7544) -> ("O/P"=w7543:string[])  [unwired: 9 in]
                      }
                      frame #6 {
                        n1372 = call "String to numeric.vi"("Array"=w7584) -> ("Array 2"=w7583:dbl[])  [unwired: 4 in]
                        n1373 = call "String to numeric.vi"("Array"=w7582) -> ("Array 2"=w7581:dbl[])  [unwired: 4 in]
                        n1374 = call "String to numeric.vi"("Array"=w7580) -> ("Array 2"=w7579:dbl[])  [unwired: 4 in]
                        n1375 = call "String to numeric.vi"("Array"=w7578) -> ("Array 2"=w7577:dbl[])  [unwired: 4 in]
                        n1376 = call "String to numeric.vi"("Array"=w7576) -> ("Array 2"=w7575:dbl[])  [unwired: 4 in]
                        n1377 = Decimal String To Number(string=w7589) -> (number=w7608:i32[])  [unwired: 2 in, 1 out]
                        n1378 = Decimal String To Number(string=w7590) -> (number=w7609:i32[])  [unwired: 2 in, 1 out]
                        n1379 = Decimal String To Number(string=w7591) -> (number=w7610:i32[])  [unwired: 2 in, 1 out]
                        n1380 = Decimal String To Number(string=w7592) -> (number=w7611:i32[])  [unwired: 2 in, 1 out]
                        n1381 = Decimal String To Number(string=w7593) -> (number=w7606:i32[])  [unwired: 2 in, 1 out]
                        n1382 = Compound Arithmetic op=ADD(w7583, w7581, w7579, w7577, w7575) -> (w7586:dbl[])
                        n1383 = Build Array(w7584) -> (w7605:string[][])
                        n1384 = Build Array(w7582) -> (w7604:string[][])
                        n1385 = Build Array(w7580) -> (w7603:string[][])
                        n1386 = Build Array(w7578) -> (w7602:string[][])
                        n1387 = Build Array(w7576) -> (w7601:string[][])
                        n1388 = Number To Fractional String(number=w7586, precision (6)=i16 2) -> (F-format string=w7585:string[])  [unwired: 2 in]
                        n1389 = Compound Arithmetic op=ADD(w7608, w7609, w7610, w7611, w7606) -> (w7612:i32[])
                        n1390 = Transpose 2D Array(2D array=w7605) -> (transposed array=w7599:string[][])
                        n1391 = Transpose 2D Array(2D array=w7604) -> (transposed array=w7598:string[][])
                        n1392 = Transpose 2D Array(2D array=w7603) -> (transposed array=w7597:string[][])
                        n1393 = Transpose 2D Array(2D array=w7602) -> (transposed array=w7596:string[][])
                        n1394 = Transpose 2D Array(2D array=w7601) -> (transposed array=w7595:string[][])
                        n1395 = Number To Decimal String(number=w7612) -> (decimal integer string=w7607:string[])  [unwired: 1 in]
                        n1396 = Build Array(w7585) -> (w7588:string[][])
                        n1397 = Transpose 2D Array(2D array=w7588) -> (transposed array=w7594:string[][])
                      }
                      frame #7 {
                        w7617 = string[] [""]
                        n1398 = Insert Into Array(array=w7625, index (col)=1 ("disabled index (col)"), new element #1=w7617, new element #2=w7617, new element #3=w7617, new element #4=w7617, new element #5=w7617, new element #6=w7617, new element #7=w7616, new element #8=w7615, new element #9=w7617, new element #10=w7617, new element #11=w7618, new element #12=w7619) -> (w7621:string[][])  [unwired: 1 in]
                        n1399 = call "flot graph for month n year.vi"("BD Date"=w7622, "error in (no error)"=w7624, "Count total"=w7618) -> ("error out"=w7623:errorcluster, "Run-Time Status"=w7620:cluster{"Array 2":timestamp[], dbl[]})  [unwired: 7 in]
                        n1400 = local write "Run-Time Status"(w7620) -> ()
                        n1401 = local write "Table"(w7621) -> ()
                      }
                    }
                  }
                  frame "all" {
                  }
                }
              }
              frame "Production" {
                n1402 = local read "Shift"() -> (w7628:string)
                n1403 = case shown="\"2\"" w7628 {
                  selector: w7628 -> [_ w8003 w8392 w8781 _]
                  tunnel: w7633 -> [w7638 w8008 w8397 w8786 _]
                  tunnel: w7632 -> [w7637 w8007 w8396 w8785 _]
                  tunnel: w7631 -> [w7636 w8006 w8395 w8784 _]
                  tunnel: w7630 -> [w7635 w8005 w8394 w8783 _]
                  tunnel: w7629 -> [w7634 w8004 w8393 w8782 _]
                  frame "ALL", Default {
                    n1404 = flat-sequence {
                      tunnel: w7638 -> [w7750]
                      tunnel: w7637 -> [w7748]
                      tunnel: [w7734] -> w7728
                      tunnel: [w7749] -> w7727
                      tunnel: w7636 -> [_]
                      tunnel: [w7753] -> w7726
                      tunnel: [w7733] -> w7725
                      tunnel: [w7732] -> w7724
                      tunnel: [w7730] -> w7723
                      tunnel: w7635 -> [w7733]
                      tunnel: w7634 -> [w7732]
                      tunnel: ["Where BREAKDOWN_DATE between '%s'and '%s' and BREAKDOWN_STK_HOLD_ID ='%d'  "] -> w7722
                      tunnel: [w7730] -> w7721
                      tunnel: w7728 -> [w7812]
                      tunnel: w7727 -> [w7814]
                      tunnel: w7726 -> [w7810]
                      tunnel: w7725 -> [w7809]
                      tunnel: w7724 -> [w7808]
                      tunnel: [w7811] -> w7720
                      tunnel: [w7813] -> w7719
                      tunnel: [w7810] -> w7718
                      tunnel: [w7800] -> w7717
                      tunnel: [w7806] -> w7716
                      tunnel: [w7809] -> w7715
                      tunnel: [w7808] -> w7714
                      tunnel: w7723 -> [w7805]
                      tunnel: [w7805] -> w7713
                      tunnel: w7722 -> [w7802]
                      tunnel: [w7802] -> w7712
                      tunnel: [w7801] -> w7711
                      tunnel: w7721 -> [w7801]
                      tunnel: w7720 -> [w7840]
                      tunnel: w7719 -> [w7838]
                      tunnel: w7718 -> [w7843]
                      tunnel: w7717 -> [w7842]
                      tunnel: w7716 -> [w7841]
                      tunnel: w7715 -> [w7836]
                      tunnel: w7714 -> [w7835]
                      tunnel: [w7843] -> w7710
                      tunnel: [w7842] -> w7709
                      tunnel: [w7841] -> w7708
                      tunnel: [w7839] -> w7707
                      tunnel: [w7833] -> w7706
                      tunnel: [w7832] -> w7705
                      tunnel: [w7837] -> w7704
                      tunnel: [w7836] -> w7703
                      tunnel: [w7835] -> w7702
                      tunnel: w7713 -> [w7831]
                      tunnel: [w7831] -> w7701
                      tunnel: w7712 -> [w7828]
                      tunnel: [w7828] -> w7700
                      tunnel: [w7827] -> w7699
                      tunnel: w7711 -> [w7827]
                      tunnel: w7710 -> [w7874]
                      tunnel: w7709 -> [w7873]
                      tunnel: w7708 -> [w7872]
                      tunnel: w7707 -> [w7869]
                      tunnel: w7706 -> [w7871]
                      tunnel: w7705 -> [w7870]
                      tunnel: w7704 -> [w7867]
                      tunnel: w7703 -> [w7865]
                      tunnel: w7702 -> [w7864]
                      tunnel: [w7874] -> w7698
                      tunnel: [w7873] -> w7697
                      tunnel: [w7872] -> w7696
                      tunnel: [w7871] -> w7695
                      tunnel: [w7870] -> w7694
                      tunnel: [w7868] -> w7693
                      tunnel: [w7862] -> w7692
                      tunnel: [w7861] -> w7691
                      tunnel: [w7866] -> w7690
                      tunnel: [w7865] -> w7689
                      tunnel: [w7864] -> w7688
                      tunnel: w7701 -> [w7860]
                      tunnel: [w7860] -> w7687
                      tunnel: w7700 -> [w7857]
                      tunnel: [w7857] -> w7686
                      tunnel: [w7856] -> w7685
                      tunnel: w7699 -> [w7856]
                      tunnel: w7698 -> [w7907]
                      tunnel: w7697 -> [w7906]
                      tunnel: w7696 -> [w7905]
                      tunnel: w7695 -> [w7904]
                      tunnel: w7694 -> [w7903]
                      tunnel: w7693 -> [w7900]
                      tunnel: w7692 -> [w7902]
                      tunnel: w7691 -> [w7901]
                      tunnel: w7690 -> [w7899]
                      tunnel: w7689 -> [w7896]
                      tunnel: w7688 -> [w7895]
                      tunnel: [w7907] -> w7684
                      tunnel: [w7906] -> w7683
                      tunnel: [w7905] -> w7682
                      tunnel: [w7904] -> w7681
                      tunnel: [w7903] -> w7680
                      tunnel: [w7902] -> w7679
                      tunnel: [w7901] -> w7678
                      tunnel: [w7898] -> w7677
                      tunnel: [w7897] -> w7676
                      tunnel: [w7893] -> w7675
                      tunnel: [w7892] -> w7674
                      tunnel: [w7896] -> w7673
                      tunnel: [w7895] -> w7672
                      tunnel: w7687 -> [w7891]
                      tunnel: [w7891] -> w7671
                      tunnel: w7686 -> [w7888]
                      tunnel: [w7888] -> w7670
                      tunnel: [w7887] -> w7669
                      tunnel: w7685 -> [w7887]
                      tunnel: w7684 -> [w7943]
                      tunnel: w7683 -> [w7942]
                      tunnel: w7682 -> [w7941]
                      tunnel: w7681 -> [w7940]
                      tunnel: w7680 -> [w7939]
                      tunnel: w7679 -> [w7938]
                      tunnel: w7678 -> [w7937]
                      tunnel: w7677 -> [w7932]
                      tunnel: w7676 -> [w7934]
                      tunnel: w7675 -> [w7936]
                      tunnel: w7674 -> [w7935]
                      tunnel: w7673 -> [w7929]
                      tunnel: w7672 -> [w7930]
                      tunnel: [w7943] -> w7668
                      tunnel: [w7942] -> w7667
                      tunnel: [w7941] -> w7666
                      tunnel: [w7940] -> w7665
                      tunnel: [w7939] -> w7664
                      tunnel: [w7938] -> w7663
                      tunnel: [w7937] -> w7662
                      tunnel: [w7936] -> w7661
                      tunnel: [w7935] -> w7660
                      tunnel: [w7933] -> w7659
                      tunnel: [w7931] -> w7658
                      tunnel: [w7927] -> w7657
                      tunnel: [w7925] -> w7656
                      tunnel: w7671 -> [w7926]
                      tunnel: w7670 -> [w7922]
                      tunnel: [w7921] -> w7655
                      tunnel: w7669 -> [w7921]
                      tunnel: w7668 -> [w7970]
                      tunnel: w7667 -> [w7963]
                      tunnel: w7666 -> [w7954]
                      tunnel: w7665 -> [w7962]
                      tunnel: w7664 -> [w7952]
                      tunnel: w7663 -> [w7961]
                      tunnel: w7662 -> [w7950]
                      tunnel: w7661 -> [w7960]
                      tunnel: w7660 -> [w7948]
                      tunnel: w7659 -> [w7984]
                      tunnel: w7658 -> [w7983]
                      tunnel: w7657 -> [w7959]
                      tunnel: w7656 -> [w7946]
                      tunnel: [w7984] -> w7654
                      tunnel: [w7983] -> w7653
                      tunnel: [w7977] -> w7652
                      tunnel: [w7970] -> w7651
                      tunnel: [w7969] -> w7650
                      tunnel: [w7968] -> w7649
                      tunnel: [w7967] -> w7648
                      tunnel: [w7966] -> w7647
                      tunnel: [w7965] -> w7646
                      tunnel: [w7964] -> w7645
                      tunnel: [w7963] -> w7644
                      tunnel: [w7962] -> w7643
                      tunnel: [w7961] -> w7642
                      tunnel: [w7960] -> w7641
                      tunnel: [w7959] -> w7640
                      tunnel: [w7944] -> w7639
                      tunnel: w7655 -> [w7944]
                      tunnel: [w7997] -> _
                      tunnel: [w7993] -> _
                      tunnel: w7654 -> [w7994]
                      tunnel: w7653 -> [w7997]
                      tunnel: w7652 -> [w7988]
                      tunnel: w7651 -> [w7995]
                      tunnel: w7650 -> [_]
                      tunnel: w7649 -> [_]
                      tunnel: w7648 -> [_]
                      tunnel: w7647 -> [_]
                      tunnel: w7646 -> [w7987]
                      tunnel: w7645 -> [w7989]
                      tunnel: w7644 -> [_]
                      tunnel: w7643 -> [_]
                      tunnel: w7642 -> [_]
                      tunnel: w7641 -> [_]
                      tunnel: w7640 -> [w7986]
                      tunnel: w7639 -> [w7992]
                      frame #0 {
                        w7741 = "%Y-%m-%d" ("time format string (%c)")
                        n1405 = property on="Table" class="Tbl (strict)"("Visible"=TRUE) -> ()  [unwired: 2 in, 2 out]
                        n1406 = Format Date/Time String(time format string (%c)=w7741, seconds (now)=w7733) -> (date/time string=w7742:string)  [unwired: 1 in]
                        n1407 = Format Date/Time String(time format string (%c)=w7741, seconds (now)=w7732) -> (date/time string=w7740:string)  [unwired: 1 in]
                        n1408 = Format Into String(format string="Where BREAKDOWN_DATE between '%s' and '%s' ", w7742, w7740) -> (resulting string=w7739:string)  [unwired: 2 in, 1 out]
                        n1409 = call <vilib>:"DB Tools Select Data.vi"("condition"=w7739, "error in (no error)"=w7748, "columns"=string[] ["BREAKDOWN_DATE"], "table"="STATION_1_LOG_HISTORY", "connection reference"=w7750) -> ("error out"=w7735:errorcluster, "data"=w7738:variant[][], "connection reference out"=w7749:T2)  [unwired: 1 in]
                        n1410 = property on="Table 2" class="Tbl (strict)"("Visible"=FALSE) -> ()  [unwired: 2 in, 2 out]
                        n1411 = xnode "Database Variant To Data"("database variant"=w7738, "error in (no error)"=w7735, "type"=string[][] [] ("Elements Found")) -> ("data"=w7736:string[][], "error out"=w7734:errorcluster)
                        n1412 = Index Array(array=w7736, index (col)=0 ("disabled index (col)")) -> (element=w7744:string[])  [unwired: 1 in]
                        n1413 = call "Search_1d_array_element.vi"("Count in"=string[] [] ("Elements Found"), "BD Date"=w7744, "Elements Found in"=string[] [] ("Elements Found")) -> ("Elements Found out"=w7730:string[])  [unwired: 4 in, 2 out]
                        n1414 = Build Array(w7730) -> (w7754:string[][])
                        n1415 = Transpose 2D Array(2D array=w7754) -> (transposed array=w7753:string[][])
                      }
                      frame #1 {
                        n1416 = disable-structure shown="Enabled" {
                          disable-tunnel: w7814 -> [w7824 w7825]
                          disable-tunnel: [w7823 w7825] -> w7813
                          disable-tunnel: w7812 -> [w7822 w7826]
                          disable-tunnel: [w7821 w7826] -> w7811
                          disable-tunnel: w7809 -> [w7819 _]
                          disable-tunnel: w7808 -> [w7818 _]
                          disable-tunnel: [w7817 _] -> w7807
                          disable-tunnel: [w7816 _] -> w7804
                          disable-tunnel: w7802 -> [w7815 _]
                          frame Disabled {
                            n1417 = call "Stack_holderwise_total_bd_count_&_duration.vi"("Refnum in"=w7824, "BREAKDOWN_STK_HOLD_ID"=1, "condition"=w7815, "Form Date"=w7819, "To Date"=w7818, "error in (no error)"=w7822) -> ("Refnum out"=w7823:T2, "Count out"=w7817:string[], "appended array"=w7816:dbl[], "error out"=w7821:errorcluster)  [unwired: 6 in]
                          }
                          frame Enabled {
                          }
                        }
                        n1418 = call "NUMERIC TO STRING.vi"("appended array"=w7804) -> ("Array"=w7803:string[])  [unwired: 4 in]
                        n1419 = call "Insert_empty_element_with_zero.vi"("searched date"=w7807, "fixed date"=w7805) -> ("O/P"=w7800:string[])  [unwired: 9 in]
                        n1420 = call "Insert_empty_element_with_zero.vi"("searched date"=w7803, "fixed date"=w7805) -> ("O/P"=w7806:string[])  [unwired: 9 in]
                      }
                      frame #2 {
                        n1421 = disable-structure shown="Enabled" {
                          disable-tunnel: w7840 -> [w7853 w7855]
                          disable-tunnel: [w7852 w7855] -> w7839
                          disable-tunnel: w7838 -> [w7851 w7854]
                          disable-tunnel: [w7850 w7854] -> w7837
                          disable-tunnel: w7836 -> [w7849 _]
                          disable-tunnel: w7835 -> [w7848 _]
                          disable-tunnel: [w7847 _] -> w7834
                          disable-tunnel: [w7846 _] -> w7830
                          disable-tunnel: w7828 -> [w7845 _]
                          frame Disabled {
                            n1422 = call "Stack_holderwise_total_bd_count_&_duration.vi"("Refnum in"=w7851, "BREAKDOWN_STK_HOLD_ID"=2, "condition"=w7845, "Form Date"=w7849, "To Date"=w7848, "error in (no error)"=w7853) -> ("Refnum out"=w7850:T2, "Count out"=w7847:string[], "appended array"=w7846:dbl[], "error out"=w7852:errorcluster)  [unwired: 6 in]
                          }
                          frame Enabled {
                          }
                        }
                        n1423 = call "Insert_empty_element_with_zero.vi"("searched date"=w7834, "fixed date"=w7831) -> ("O/P"=w7833:string[])  [unwired: 9 in]
                        n1424 = call "NUMERIC TO STRING.vi"("appended array"=w7830) -> ("Array"=w7829:string[])  [unwired: 4 in]
                        n1425 = call "Insert_empty_element_with_zero.vi"("searched date"=w7829, "fixed date"=w7831) -> ("O/P"=w7832:string[])  [unwired: 9 in]
                      }
                      frame #3 {
                        n1426 = disable-structure shown="Enabled" {
                          disable-tunnel: w7869 -> [w7884 w7886]
                          disable-tunnel: [w7883 w7886] -> w7868
                          disable-tunnel: w7867 -> [w7882 w7885]
                          disable-tunnel: [w7881 w7885] -> w7866
                          disable-tunnel: w7865 -> [w7880 _]
                          disable-tunnel: w7864 -> [w7879 _]
                          disable-tunnel: [w7878 _] -> w7863
                          disable-tunnel: [w7877 _] -> w7859
                          disable-tunnel: w7857 -> [w7876 _]
                          frame Disabled {
                            n1427 = call "Stack_holderwise_total_bd_count_&_duration.vi"("Refnum in"=w7882, "BREAKDOWN_STK_HOLD_ID"=3, "condition"=w7876, "Form Date"=w7880, "To Date"=w7879, "error in (no error)"=w7884) -> ("Refnum out"=w7881:T2, "Count out"=w7878:string[], "appended array"=w7877:dbl[], "error out"=w7883:errorcluster)  [unwired: 6 in]
                          }
                          frame Enabled {
                          }
                        }
                        n1428 = call "Insert_empty_element_with_zero.vi"("searched date"=w7863, "fixed date"=w7860) -> ("O/P"=w7862:string[])  [unwired: 9 in]
                        n1429 = call "NUMERIC TO STRING.vi"("appended array"=w7859) -> ("Array"=w7858:string[])  [unwired: 4 in]
                        n1430 = call "Insert_empty_element_with_zero.vi"("searched date"=w7858, "fixed date"=w7860) -> ("O/P"=w7861:string[])  [unwired: 9 in]
                      }
                      frame #4 {
                        n1431 = disable-structure shown="Enabled" {
                          disable-tunnel: w7900 -> [w7917 w7919]
                          disable-tunnel: w7899 -> [w7916 w7918]
                          disable-tunnel: [w7915 w7918] -> w7898
                          disable-tunnel: [w7914 w7919] -> w7897
                          disable-tunnel: w7896 -> [w7913 _]
                          disable-tunnel: w7895 -> [w7912 _]
                          disable-tunnel: [w7911 _] -> w7894
                          disable-tunnel: [w7910 _] -> w7890
                          disable-tunnel: w7888 -> [w7909 _]
                          frame Disabled {
                            n1432 = call "Stack_holderwise_total_bd_count_&_duration.vi"("Refnum in"=w7916, "BREAKDOWN_STK_HOLD_ID"=4, "condition"=w7909, "Form Date"=w7913, "To Date"=w7912, "error in (no error)"=w7917) -> ("Refnum out"=w7915:T2, "Count out"=w7911:string[], "appended array"=w7910:dbl[], "error out"=w7914:errorcluster)  [unwired: 6 in]
                          }
                          frame Enabled {
                          }
                        }
                        n1433 = call "Insert_empty_element_with_zero.vi"("searched date"=w7894, "fixed date"=w7891) -> ("O/P"=w7893:string[])  [unwired: 9 in]
                        n1434 = call "NUMERIC TO STRING.vi"("appended array"=w7890) -> ("Array"=w7889:string[])  [unwired: 4 in]
                        n1435 = call "Insert_empty_element_with_zero.vi"("searched date"=w7889, "fixed date"=w7891) -> ("O/P"=w7892:string[])  [unwired: 9 in]
                      }
                      frame #5 {
                        n1436 = call "Stack_holderwise_total_bd_count_&_duration.vi"("Refnum in"=w7932, "BREAKDOWN_STK_HOLD_ID"=5, "condition"=w7922, "Form Date"=w7929, "To Date"=w7930, "error in (no error)"=w7934) -> ("Refnum out"=w7931:T2, "Count out"=w7928:string[], "appended array"=w7924:dbl[], "error out"=w7933:errorcluster)  [unwired: 6 in]
                        n1437 = call "NUMERIC TO STRING.vi"("appended array"=w7924) -> ("Array"=w7923:string[])  [unwired: 4 in]
                        n1438 = call "Insert_empty_element_with_zero.vi"("searched date"=w7928, "fixed date"=w7926) -> ("O/P"=w7927:string[])  [unwired: 9 in]
                        n1439 = call "Insert_empty_element_with_zero.vi"("searched date"=w7923, "fixed date"=w7926) -> ("O/P"=w7925:string[])  [unwired: 9 in]
                      }
                      frame #6 {
                        n1440 = call "String to numeric.vi"("Array"=w7954) -> ("Array 2"=w7953:dbl[])  [unwired: 4 in]
                        n1441 = call "String to numeric.vi"("Array"=w7952) -> ("Array 2"=w7951:dbl[])  [unwired: 4 in]
                        n1442 = call "String to numeric.vi"("Array"=w7950) -> ("Array 2"=w7949:dbl[])  [unwired: 4 in]
                        n1443 = call "String to numeric.vi"("Array"=w7948) -> ("Array 2"=w7947:dbl[])  [unwired: 4 in]
                        n1444 = call "String to numeric.vi"("Array"=w7946) -> ("Array 2"=w7945:dbl[])  [unwired: 4 in]
                        n1445 = Decimal String To Number(string=w7959) -> (number=w7978:i32[])  [unwired: 2 in, 1 out]
                        n1446 = Decimal String To Number(string=w7960) -> (number=w7979:i32[])  [unwired: 2 in, 1 out]
                        n1447 = Decimal String To Number(string=w7961) -> (number=w7980:i32[])  [unwired: 2 in, 1 out]
                        n1448 = Decimal String To Number(string=w7962) -> (number=w7981:i32[])  [unwired: 2 in, 1 out]
                        n1449 = Decimal String To Number(string=w7963) -> (number=w7976:i32[])  [unwired: 2 in, 1 out]
                        n1450 = Compound Arithmetic op=ADD(w7953, w7951, w7949, w7947, w7945) -> (w7956:dbl[])
                        n1451 = Build Array(w7954) -> (w7975:string[][])
                        n1452 = Build Array(w7952) -> (w7974:string[][])
                        n1453 = Build Array(w7950) -> (w7973:string[][])
                        n1454 = Build Array(w7948) -> (w7972:string[][])
                        n1455 = Build Array(w7946) -> (w7971:string[][])
                        n1456 = Number To Fractional String(number=w7956, precision (6)=i16 2) -> (F-format string=w7955:string[])  [unwired: 2 in]
                        n1457 = Compound Arithmetic op=ADD(w7978, w7979, w7980, w7981, w7976) -> (w7982:i32[])
                        n1458 = Transpose 2D Array(2D array=w7975) -> (transposed array=w7969:string[][])
                        n1459 = Transpose 2D Array(2D array=w7974) -> (transposed array=w7968:string[][])
                        n1460 = Transpose 2D Array(2D array=w7973) -> (transposed array=w7967:string[][])
                        n1461 = Transpose 2D Array(2D array=w7972) -> (transposed array=w7966:string[][])
